vi "Puma_Ground_Control_Station_V2.0.vi"(0 "?":refnum<visa-resource-name>="COM3", 1 "?":u32=9600, 9 "XON":u8=17 format="%.0x", 14 "XOFF":u8=19 format="%.0x", 15 "?":u32=10000, 21 "?":bool=TRUE, 24 "?":u8=10 format="%.0x", 25 "bsize":u32=4096) -> ()   [LabVIEW 2015]
doc: "The Advanced Serial Read and Write example performs a Serial Port Read, a Serial Port Write, or a combination of these actions while setting some advanced serial features like buffer size, termination characters, and XON/XOFF flow control. The user selects the actions (read or write) on the front panel. If both are selected, the VI will write the data first, read the data and then close the VISA session that is opened to the port. \n\nThe parameters set for the serial port must match the parameters of the connected instrument or device. In this example, the bytes to read parameter specifies the number of bytes that the serial port reads. If there were more bytes at the port than the number specified in bytes to read, those bytes would not be read. Also, if you specify to read more bytes than the number of bytes actually read, you might receive a timeout error message.\n\nINSTRUCTIONS:\n1) Select the serial resource and configuration parameters (baud rate, data bits, parity, stop bits, flow control).\n2) Termination character can be enabled and set. Also, set the required input buffer size prior to running the example.\n3) Select the operations to be performed. \n4) Connect the serial port to your device. If no device is available, perform a loopback test by doing one of the following. Short pins 2 and 3 on a RS-232 cable or short pin 4 to pin 8 and pin 5 to pin 9 on a RS-485/422 cable. \n5) Run the VI to see the data read. (The \"read string\" will match the \"string to write\" if a loopback test was performed.)\n\nThis example exposes several advanced features that you may need for your application. Not all applications need all the features shown in this example. The input buffer size is likely an important setting that you want to control in your application. This example expands upon the flow control option for XON and XOFF, allowing the user to choose those control characters. The timeout parameter has been brought to the front panel so a user can specify the time period the VISA Read will wait for the number of bytes to read before timing out. Also, the user has several controls for the termination character, which is discussed later.\n\nNote that you can press the write and read buttons and change the bytes to read parameters on the fly, while the example is running. However, you must stop the example to change the other configuration parameters after the example has started running, and then run again.\n\nSet the I/O buffer size slightly higher the amount of data you expect to receive. This is very important for applications that don't use flow control, as you may lose characters if the receive buffer overflows.\n\nSetting the timeout period ensures that the operation returns with a timeout error if the operation cannot be performed in the specified time period. \n\nSome devices require a termination character in order to identify the end of command strings. Some devices send a termination character to signify the end of data to be read. \n\nThis example shows how you can end the Read operation once a termination character is detected in the buffer and/or append a termination character at the end of the Write data. To enable the Read to end on a termination character, use the VISA Configure Serial Port or use the VISA Properties Serial End Mode for Reads, Termination Character Enable, and Termination Character. To end the Write with a termination character, use the VISA Properties Serial End Mode for Writes, the Send End Enable, and Termination Character. In this example, the same termination character is used for both the Read and the Write. You can specify two different characters for your application, if desired.\n\nYour application may require specific characters for the XON/XOFF Flow Control. You can specify these characters with the VISA Properties Flow Control XOFF Character and Flow Control XON Character. Note that if the standard XON and XOFF characters are used, then decimal 17 and 19 are unavailable for data values. Remember that using flow control and setting an adequate buffer size allow you to prevent buffer overflows."
uses:
  <vilib>/Instr/_visa.llb/VISA Configure Serial Port (Instr).vi
panel:
  out "Numeric":i32
  out "Reset Triggered":bool
  in  "PixHawk":bool
  in  "XON 2":u8=17 format="%.0x"
  in  "XOFF 2":u8=19 format="%.0x"
  in  "?":bool=TRUE
  in  "bsize 2":u32=4096
  in  "?":u8=10 format="%.0x"
  in  "?":bool=TRUE
  in  "?":u32=10000
  in  "?":refnum<visa-resource-name>="COM3"
  in  "?":u32=9600
  out "Max Values":T1={20.764332288, 0.0, 0.0, 0.0, 0.0, 0.0, 0.0, 201.058, 25.138999999999953, 0.0, 57.16000000000008, 0.0, 8.920000000000016, 15.403999999999996}
  in  "Data Filename":string
  out "Offset 7":dbl=-251.3
  out "Multiplier 7":dbl=1.264
  out "Offset 6":dbl=-250.2
  out "Offset 5":dbl=-250.3
  out "Offset 4":dbl=-1253.0
  out "Offset 3":dbl=-250.9
  out "Offset 2":dbl=-249.8
  out "Offset 1":dbl=-251.0
  out "Multiplier 6":dbl=1.264
  out "Multiplier 5":dbl=1.277
  out "Multiplier 4":dbl=6.36
  out "Multiplier 3":dbl=1.274
  out "Multiplier 2":dbl=1.267
  out "Multiplier 1":dbl=1.277
  out "Ready to Test":bool
  out "AV5-T Open":bool
  in  "Begin Checklist":bool
  out "Manual Abort Tested":bool
  out "Flight Control On":bool
  out "Reset Triggered 2":bool
  out "Primary Safety Active":bool
  out "Craft Triggered Softkill Active":bool
  out "Hardkill Active":bool
  out "ms":dbl=163640.0
  out "vcc 6":bool
  out "gnd 6":bool=TRUE
  out "TC6":bool
  out "vcc 5":bool
  out "gnd 5":bool=TRUE
  out "TC5":bool
  out "vcc 4":bool
  out "gnd 4":bool=TRUE
  out "TC4":bool
  out "vcc 3":bool
  out "gnd 3":bool=TRUE
  out "TC3":bool
  out "vcc 2":bool
  out "gnd 2":bool=TRUE
  out "TC2":bool
  out "vcc":bool
  out "gnd":bool=TRUE
  out "TC1":bool
  out "Motor 4":dbl=1000.0
  out "Motor 3":dbl=1000.0
  out "Motor 2":dbl=1000.0
  out "Motor 1":dbl=1000.0
  out "soft kill ind":bool
  out "dump fuel ind":bool
  out "abort ind":bool
  out "run ind":bool
  out "av6-t ind":bool
  out "Control input":bool
  out "return":bool
  out "Control (on/off)":bool
  out "PT5-M":dbl=-6.084000000000003
  out "PT2-M":dbl=-10.039999999999992
  out "PT2-U":dbl=-250.3
  out "PT1-U":dbl=-38.24000000000001
  out "PT3-M":dbl=-141.336
  out "PT1-M":dbl=9.934999999999945
  out "PT4-M":dbl=181.90299999999996
  out "TC6":dbl=-2.0
  out "TC5":dbl=-2.0
  out "TC4":dbl=-2.0
  out "TC3":dbl=-2.0
  out "TC2":dbl=-2.0
  out "TC1":dbl=-2.0
  out "Output":string="h:;"
  in  "?":enum32{"Ignore", "Test"}(tab)=enum."Test"
  in  "DValve / AV6-T":bool
  in  "Flight Control Board":bool
  in  "Safety":bool
  in  "Test Run":bool
  in  "Reset Control":bool
  in  "Primary Safety":bool
  out "?":bool
  in  "Primary Safety":bool=TRUE
  in  "Soft Kill":bool
  in  "Simulate":bool
  in  "Reset FC":bool
  in  "Full Power":bool
  in  "Safety":bool=TRUE
  in  "Takeoff":bool
  in  "Calibrate":bool
  in  "abort":bool
  out "?":dbl(graph)=20.40794784
  in  "Send":bool=TRUE
  in  "Recieve":bool=TRUE
  in  "bytes to read 2":u32=1000
  out "?":u32=107
  out "?":string[](array[string])=["339", "205", "86", "191", "0", "190", "194", "-2.00", "-2.00", "-2.00", "-2.00", "-2.00", "-2.00", "555", "1000", "1000", "1000", "1000", "163640"]
  out "?":string[](array[string])=["p:339,205,86,191,0,190,194", "t:-2.00,-2.00,-2.00,-2.00,-2.00,-2.00", "v:555", "m:1000,1000,1000,1000", "h:", "s:163640", ""]
  out "?":T1(graph)={20.40794784, -2.0, -2.0, -2.0, -2.0, -2.0, -2.0, 181.90299999999996, 9.934999999999945, -141.336, -38.24000000000001, -250.3, -10.039999999999992, -6.084000000000003}
  out "Voltage Sensor":dbl=20.40794784
  in  "dump fuel":bool
  in  "?":enum32{"PT", "TC", "Motors", "Ignore"}(tab)
  in  "?":T2(tab)
  out "PT 4":dbl(graph)=-38.24000000000001
  out "PT 5":dbl(graph)=-250.3
  out "PT 2":dbl(graph)=9.934999999999945
  out "PT 6":dbl(graph)=-10.039999999999992
  out "PT 3":dbl(graph)=-141.336
  out "PT 1":dbl(graph)=181.90299999999996
  out "PT 7":dbl(graph)=-6.084000000000003
  in  "?":T3(tab)
  out "TC 1":dbl(graph)=-2.0
  out "TC 2":dbl(graph)=-2.0
  out "TC 3":dbl(graph)=-2.0
  out "TC 4":dbl(graph)=-2.0
  out "TC 5":dbl(graph)=-2.0
  out "TC 6":dbl(graph)=-2.0
  out "Motors":cluster{dbl, dbl, dbl, dbl}(graph)={1000.0, 1000.0, 1000.0, 1000.0}
  out "?":bool=TRUE
  out "String":string
  in  "String 3":string
  in  "?":bool=TRUE
  in  "tank iso":bool
  in  "Av-6Tt":bool
  in  "FC-U Toggle":bool
  in  "FOU":bool
  out "AV4-T":bool
  out "AV3-T":bool
  out "AV2-T":bool
  out "AV1-T":bool
  out "AV6-T":bool
  out "AV5-T":bool
  out "FO-U":bool
  out "FC-U":bool
  out "?":dbl(slide) scale=0.2..200.0
  # "green=open - check thermocouple attachments\nred=short gnd - contact Power or GNC\nblue=short vcc - contact Power or GNC"
  # "String Parsing Indicator"
  # "Data From Craft:"
  # "FC-U"
  # "FO-U"
  # "receive"
  # "AV1-M"
  # "AV2-M"
  # "AV3-M"
  # "AV4-M"
  # "AV5-T"
  # "send"
  # "AV6-T"
  # "Voltage"
  # "TCp2-M"
  # "Tcw1-E"
  # "TCp1-M"
  # "TCw4-E"
  # "TCw3-E"
  # "TCw2-E"
  # "PT4-M"
  # "PT1-M"
  # "PT3-M"
  # "PT1-U"
  # "PT2-U"
  # "PT2-M"
  # "PT5-M"
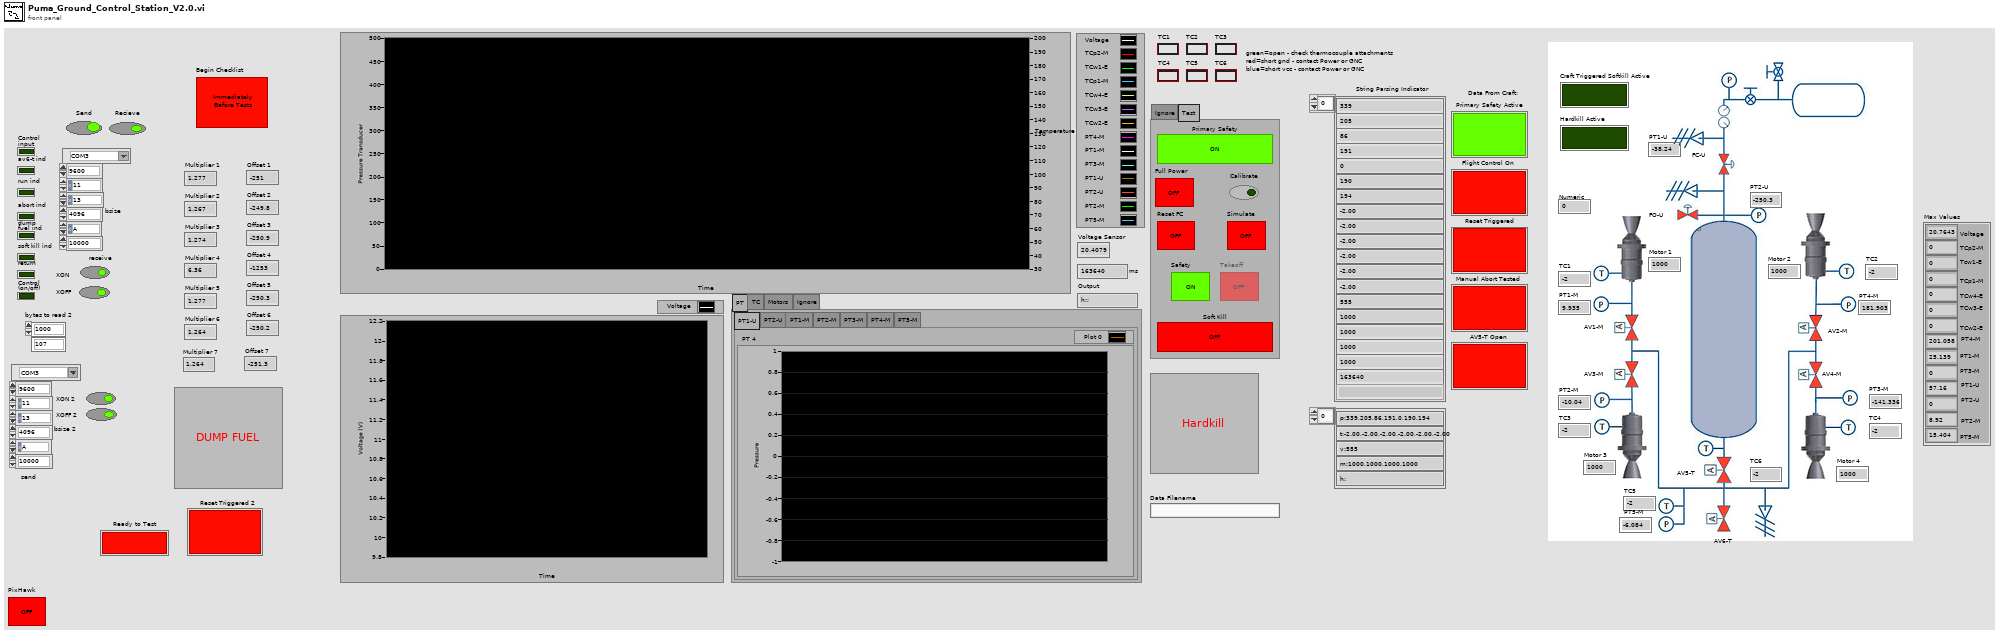
[diagram p1: front panel]
types:
  T1 = cluster{dbl, dbl, dbl, dbl, dbl, dbl, dbl, dbl, dbl, dbl, dbl, dbl, dbl, dbl}
  T2 = enum32{"PT1-U", "PT2-U", "PT1-M", "PT2-M", "PT3-M", "PT4-M", "PT5-M"}
  T3 = enum32{"TCp2-M", "TCw1-E", "TCp1-M", "TCw4-E", "TCw3-E", "TCw2-E"}
  T4 = enum16{"open", "replace", "create", "open or create", "replace or create", "replace or create with confirmation"}
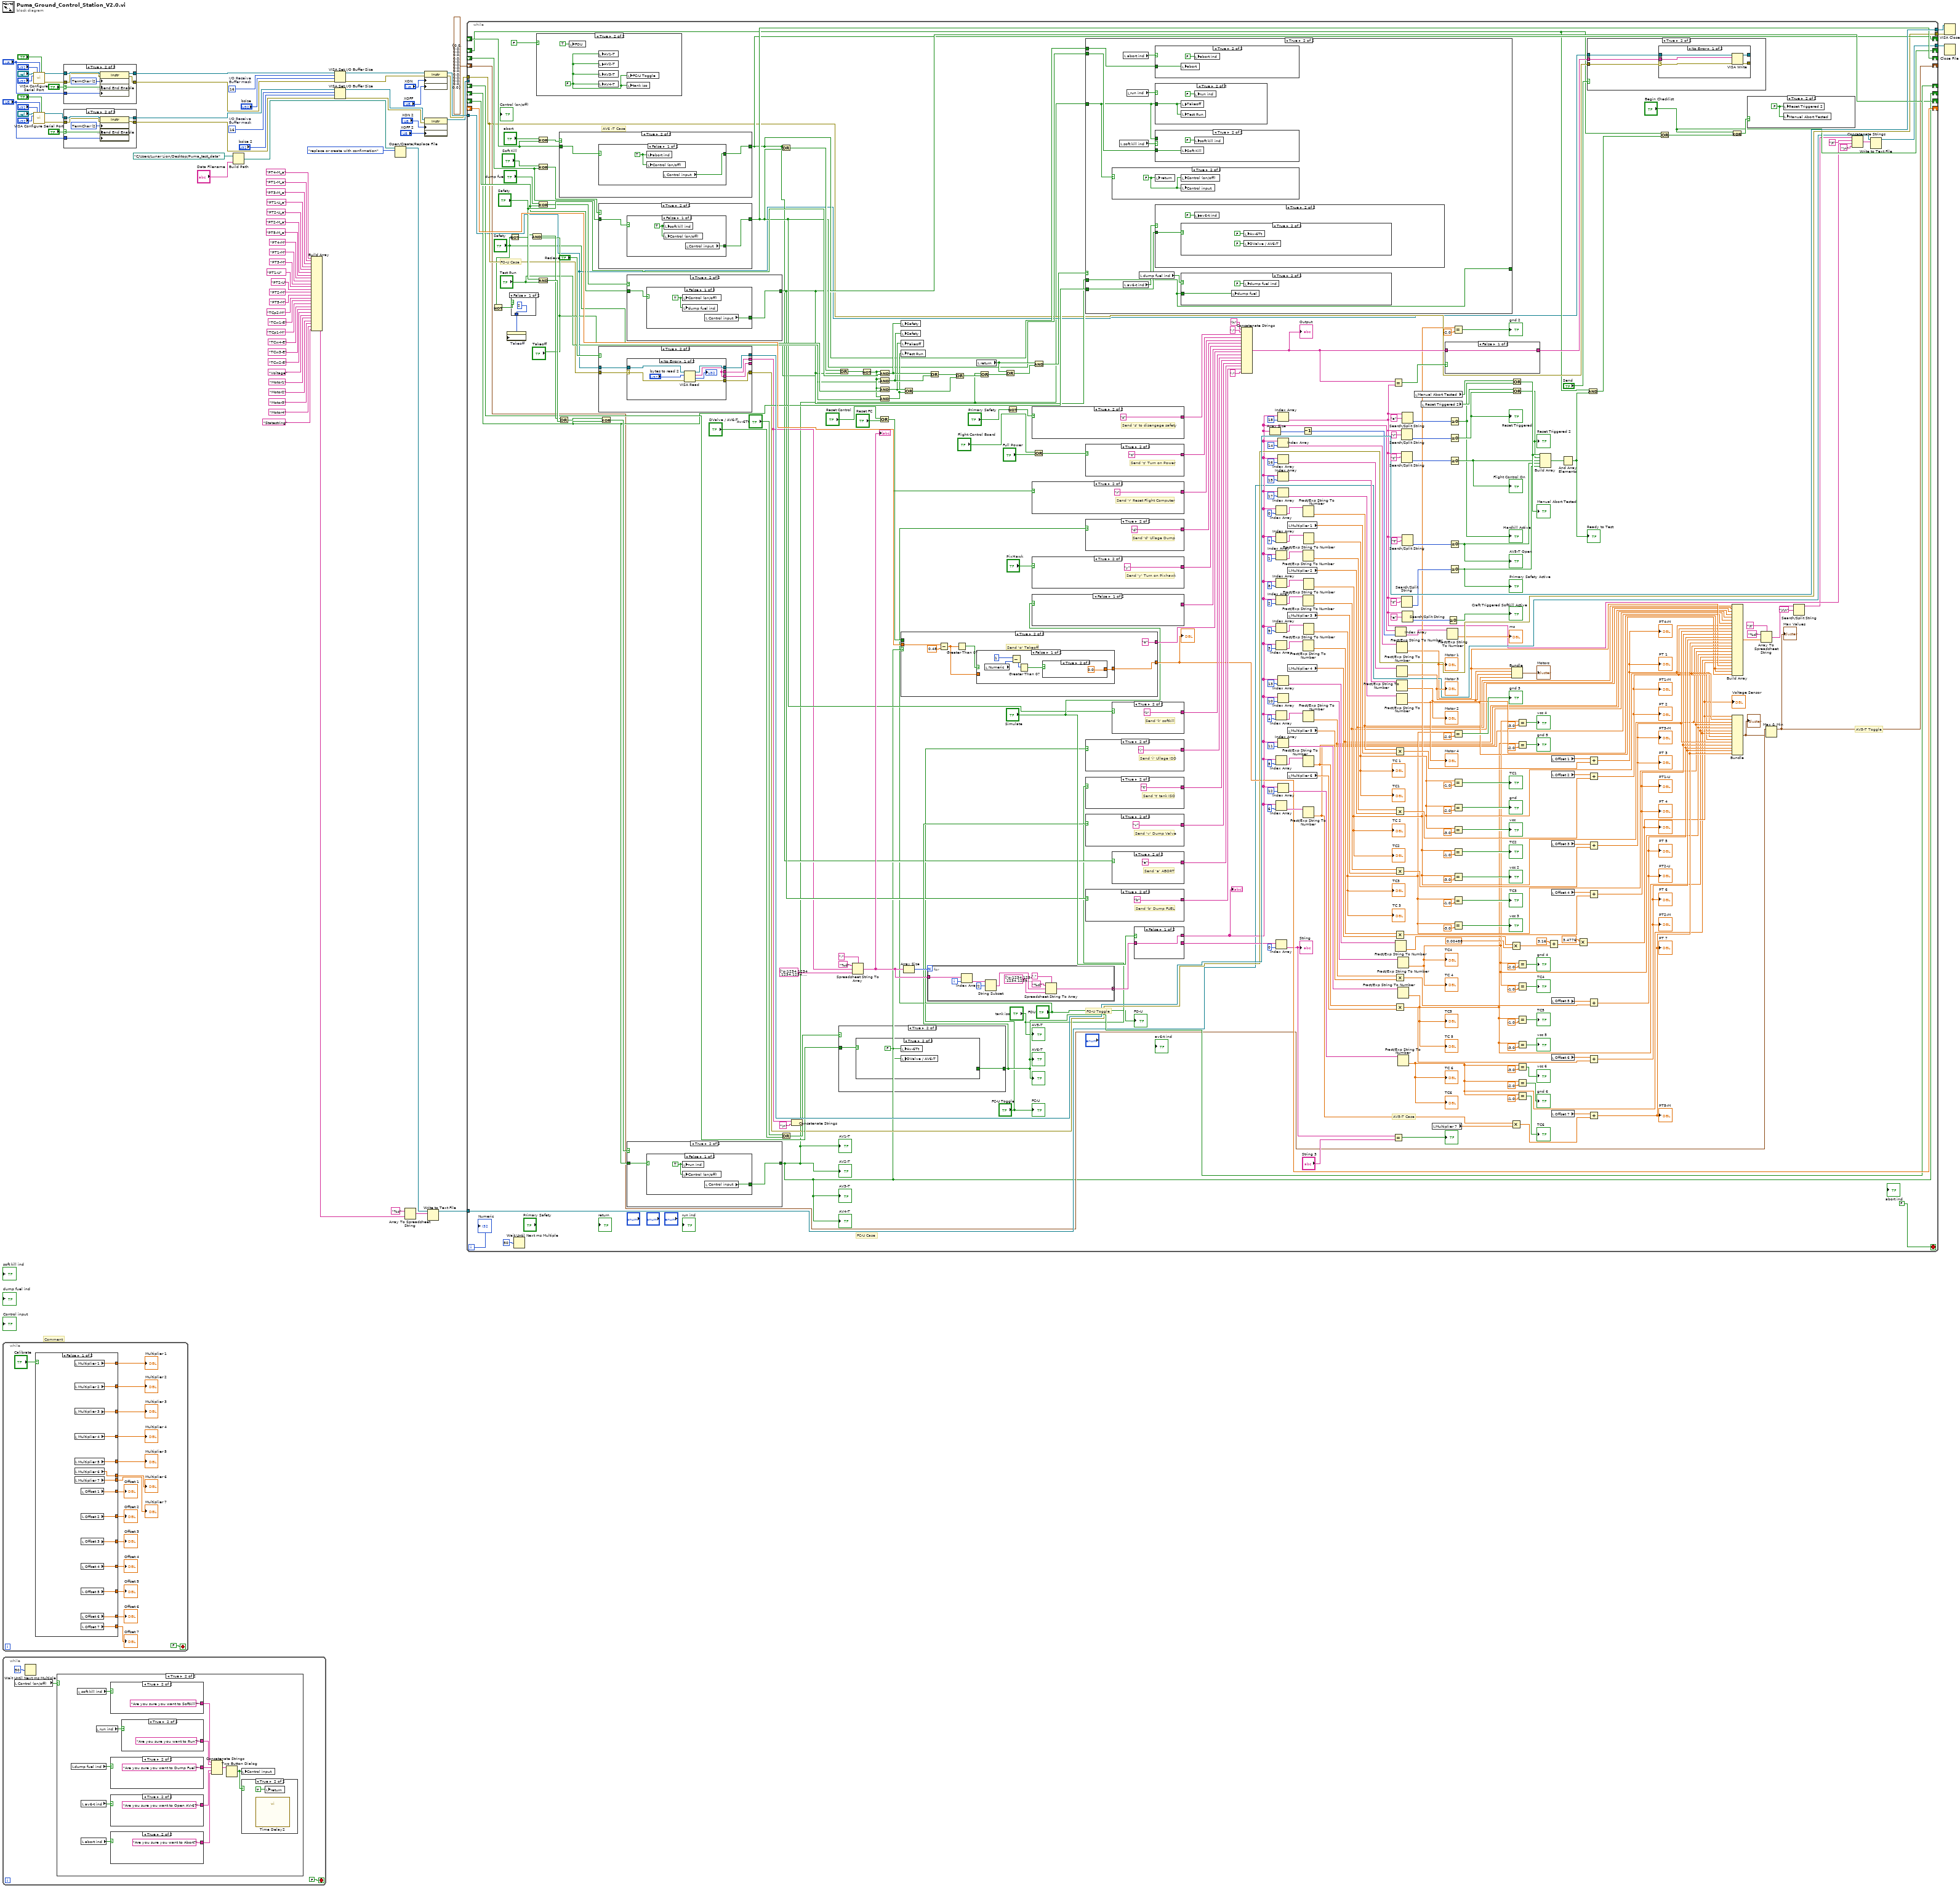
[diagram p0: block diagram]
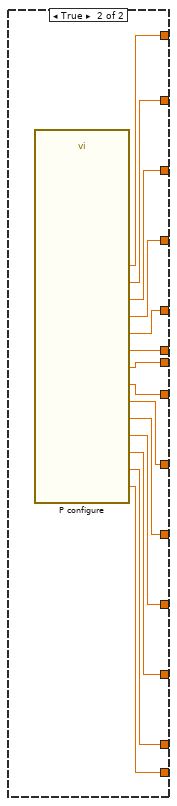
[diagram p3: hidden frame]
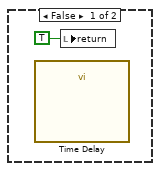
[diagram p10: hidden frame]
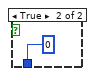
[diagram p11: hidden frame]
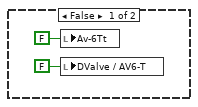
[diagram p17: hidden frame]
diagram:
  w45 = u16 16  # I/O Receive Buffer mask
  w70 = u16 16  # I/O Receive Buffer mask
  # "Comment"
  n1 = while {
    stop <- FALSE stop-if-true
    n2 = case shown="False" "Calibrate" {
      tunnel: [w104 w118] -> w88
      tunnel: [w103 w117] -> w87
      tunnel: [w102 w116] -> w86
      tunnel: [w101 w115] -> w85
      tunnel: [w100 w114] -> w84
      tunnel: [w99 w113] -> w83
      tunnel: [w98 w112] -> w82
      tunnel: [w96 w111] -> w81
      tunnel: [w97 w110] -> w80
      tunnel: [w95 w109] -> w79
      tunnel: [w94 w108] -> w78
      tunnel: [w93 w107] -> w77
      tunnel: [w92 w106] -> w76
      tunnel: [w91 w105] -> w75
      frame False {
        n3 = local read "Multiplier 1"() -> (w104:dbl)
        n4 = local read "Multiplier 2"() -> (w103:dbl)
        n5 = local read "Multiplier 3"() -> (w102:dbl)
        n6 = local read "Multiplier 4"() -> (w101:dbl)
        n7 = local read "Multiplier 5"() -> (w100:dbl)
        n8 = local read "Multiplier 6"() -> (w99:dbl)
        n9 = local read "Multiplier 7"() -> (w98:dbl)
        n10 = local read "Offset 1"() -> (w96:dbl)
        n11 = local read "Offset 2"() -> (w97:dbl)
        n12 = local read "Offset 3"() -> (w95:dbl)
        n13 = local read "Offset 4"() -> (w94:dbl)
        n14 = local read "Offset 5"() -> (w93:dbl)
        n15 = local read "Offset 6"() -> (w92:dbl)
        n16 = local read "Offset 7"() -> (w91:dbl)
      }
      frame True {
        n17 = call "P configure.vi"() -> ("Multiplier 1"=w118:dbl, "Offset 1"=w111:dbl, "Multiplier 2"=w117:dbl, "Offset 2"=w110:dbl, "Multiplier 3"=w116:dbl, "Offset 6"=w106:dbl, "Offset 3"=w109:dbl, "Offset 7"=w105:dbl, "Multiplier 4"=w115:dbl, "Multiplier 7"=w112:dbl, "Multiplier 6"=w113:dbl, "Offset 5"=w107:dbl, "Multiplier 5"=w114:dbl, "Offset 4"=w108:dbl)  [unwired: 2 in]
      }
    }
    "Multiplier 1" <- w88
    "Multiplier 2" <- w87
    "Multiplier 3" <- w86
    "Multiplier 4" <- w85
    "Multiplier 5" <- w84
    "Offset 1" <- w81
    "Offset 2" <- w80
    "Offset 3" <- w79
    "Offset 4" <- w78
    "Offset 5" <- w77
    "Offset 6" <- w76
    "Multiplier 7" <- w82
    "Offset 7" <- w75
    "Multiplier 6" <- w83
  }
  n18 = while {
    stop <- FALSE stop-if-true
    n19 = local read "Control (on/off)"() -> (w121:bool)
    n20 = Wait Until Next ms Multiple(millisecond multiple=u32 50 ("milliseconds to wait")) -> ()  [unwired: 1 out]
    n21 = case shown="True" w121 {
      frame False {
      }
      frame True {
        n22 = local read "dump fuel ind"() -> (w130:bool)
        n23 = local read "soft kill ind"() -> (w128:bool)
        n24 = local read "av6-t ind"() -> (w131:bool)
        n25 = local read "abort ind"() -> (w132:bool)
        n26 = local read "run ind"() -> (w129:bool)
        n27 = case shown="True" w128 {
          tunnel: [_ "Are you sure you want to Softkill?"] -> w123
          frame False {
          }
          frame True {
          }
        }
        n28 = case shown="True" w130 {
          tunnel: [_ "Are you sure you want to Dump Fuel?"] -> w125
          frame False {
          }
          frame True {
          }
        }
        n29 = case shown="True" w131 {
          tunnel: [_ "Are you sure you want to Open AV-6?"] -> w126
          frame False {
          }
          frame True {
          }
        }
        n30 = case shown="True" w132 {
          tunnel: [_ "Are you sure you want to Abort?"] -> w127
          frame False {
          }
          frame True {
          }
        }
        n31 = case shown="True" w129 {
          tunnel: [_ "Are you sure you want to Run?"] -> w124
          frame False {
          }
          frame True {
          }
        }
        n32 = Concatenate Strings(w123, w124, w125, w126, w127) -> (w122:string)
        n33 = Two Button Dialog(message=w122) -> (T button?=w133:bool)  [unwired: 2 in]
        n34 = local write "Control input"(w133) -> ()
        n35 = case shown="True" w133 {
          frame False {
            n36 = call "Time Delay"() -> ()  [unwired: 11 in, 1 out]
            n37 = local write "return"(TRUE) -> ()
          }
          frame True {
            n38 = call "Time Delay2"() -> ()  [unwired: 11 in, 1 out]
            n39 = local write "return"(TRUE) -> ()
          }
        }
      }
    }
  }
  n40 = call-poly "VISA Configure Serial Port"("VISA resource name"="?", "timeout (10sec)"="?", "termination char\n(0xA = '\\n' = LF)"="?", "Enable Termination\nChar (T)"="?", "baud rate (9600)"="?") -> ("VISA resource name out"=w59:refnum<visa-resource-name>, "error out"=w62:errorcluster)  [unwired: 5 in, 4 out]
  n41 = call-poly "VISA Configure Serial Port"("VISA resource name"="?", "timeout (10sec)"="?", "termination char\n(0xA = '\\n' = LF)"="?", "Enable Termination\nChar (T)"="?", "baud rate (9600)"="?") -> ("VISA resource name out"=w34:refnum<visa-resource-name>, "error out"=w37:errorcluster)  [unwired: 5 in, 4 out]
  n42 = case shown="True" "?" {
    selector: "?" -> [_ w143]
    tunnel: w59 -> [w141 w149]
    tunnel: w62 -> [w142 w148]
    tunnel: [w141 w147] -> w60
    tunnel: [w142 w146] -> w61
    tunnel: "?" -> [_ w144]
    frame False {
    }
    frame True {
      w145 = u16 2 items=["None", "LastBit", "TermChar", "Break"] ("Serial Settings:Serial End Mode for Writes")
      n43 = property class="Instr"(reference=w149, error in=w148, "Serial Settings:End Mode for Writes"=w145, "Message Based Settings:Send End Enable"=w143, "Message Based Settings:Termination Character"=w144) -> (reference out=w147:refnum<visa-resource-name>, error out=w146:errorcluster)
    }
  }
  n44 = case shown="True" "?" {
    selector: "?" -> [_ w152]
    tunnel: w34 -> [w150 w158]
    tunnel: w37 -> [w151 w157]
    tunnel: [w150 w156] -> w35
    tunnel: [w151 w155] -> w36
    tunnel: "?" -> [_ w153]
    frame False {
    }
    frame True {
      w154 = u16 2 items=["None", "LastBit", "TermChar", "Break"] ("Serial Settings:Serial End Mode for Writes")
      n45 = property class="Instr"(reference=w158, error in=w157, "Serial Settings:End Mode for Writes"=w154, "Message Based Settings:Send End Enable"=w152, "Message Based Settings:Termination Character"=w153) -> (reference out=w156:refnum<visa-resource-name>, error out=w155:errorcluster)
    }
  }
  n46 = Build Path(base path=path "C:/Users/Lunar Lion/Desktop/Puma_test_data" ("file path (use dialog)"), name or relative path="Data Filename") -> (appended path=w53:path)
  n47 = Build Array("PT4-M_a", "PT1-M_a", "PT3-M_a", "PT1-U_a", "PT2-U_a", "PT2-M_a", "PT5-M_a", "PT4-M", "PT1-M", "PT3-M", "PT1-U", "PT2-U", "PT2-M", "PT5-M", "TCp2-M", "TCw1-E", "TCp1-M", "TCw4-E", "TCw3-E", "TCw2-E", "Voltage", "Motor1", "Motor2", "Motor3", "Motor4", "Statestring") -> (w6:string[])
  n48 = VISA Set I/O Buffer Size(VISA resource name=w60, mask (16)=w70, size (4096)="bsize", error in (no error)=w61) -> (VISA resource name out=w66:refnum<visa-resource-name>, error out=w65:errorcluster)
  n49 = VISA Set I/O Buffer Size(VISA resource name=w35, mask (16)=w45, size (4096)="bsize 2", error in (no error)=w36) -> (VISA resource name out=w41:refnum<visa-resource-name>, error out=w40:errorcluster)
  n50 = Open/Create/Replace File(file path (use dialog)=w53, operation (0:open)=T4."replace or create with confirmation") -> (refnum out=w3:refnum<file>)  [unwired: 4 in, 2 out]
  n51 = Array To Spreadsheet String(array=w6, 3:"%s" ("format string")) -> (spreadsheet string=w4:string)  [unwired: 1 in]
  n52 = property class="Instr"(reference=w66, error in=w65, "Serial Settings:Flow Control XON Character"="XON", "Serial Settings:Flow Control XOFF Character"="XOFF") -> (reference out=w58:refnum<visa-resource-name>, error out=w57:errorcluster)
  n53 = property class="Instr"(reference=w41, error in=w40, "Serial Settings:Flow Control XON Character"="XON 2", "Serial Settings:Flow Control XOFF Character"="XOFF 2") -> (reference out=w33:refnum<visa-resource-name>)  [unwired: 1 out]
  n54 = Write to Text File(file (use dialog)=w3, text=w4) -> (refnum out=w2:refnum<file>)  [unwired: 2 in, 2 out]
  n55 = while {
    tunnel: w58 -> [w187]
    tunnel: w57 -> [w267]
    tunnel: [w403] -> w1
    tunnel: [w329] -> w56
    shift-right: [w375] -> _
    shift-left: _ -> [w374]
    shift-right: [w186] -> _
    shift-left: _ -> [w333]
    shift-right: [w341] -> _
    shift-left: _ -> [w342]
    shift-right: [w331] -> _
    shift-left: _ -> [w357]
    shift-right: [w332] -> _
    shift-left: _ -> [w354]
    shift-right: [w334] -> _
    shift-left: _ -> [w337]
    shift-right: ["Begin Checklist"] -> _
    shift-left: _ -> [w248]
    tunnel: w2 -> [w220]
    tunnel: [w217] -> w52
    shift-right: [w190] -> _
    shift-left: T1 {0.0, 0.0, 0.0, 0.0, 0.0, 0.0, 0.0, 0.0, 0.0, 0.0, 0.0, 0.0, 0.0, 0.0} -> [w189]
    tunnel: w33 -> [_]
    i -> [w159]
    stop <- FALSE stop-if-true
    # "FO-U Case"
    # "AV6 -T Case"
    # "AV5-T Case"
    # "FC-U Case"
    # "FO-U Toggle"
    # "AV5-T Toggle"
    n56 = Not(x="Safety") -> (.not. x?=w162:bool)
    n57 = Not(x="Safety") -> (.not. x?=w160:bool)
    n58 = case shown="False" w162 {
      tunnel: [2 0] -> w161
      frame False {
      }
      frame True {
      }
    }
    n59 = property on="Takeoff" class="Bool (strict)"("DisabledEnum"=w161) -> ()  [unwired: 2 in, 2 out]
    n60 = Wait Until Next ms Multiple(millisecond multiple=u32 50 ("milliseconds to wait")) -> ()  [unwired: 1 out]
    n61 = And(x=w160, y="Takeoff") -> (x .and. y?=w389:bool)
    n62 = case shown="True" FALSE {
      frame False {
      }
      frame True {
        w437 = FALSE
        n63 = local write "FOU"(TRUE) -> ()
        n64 = local write "AV1-T"(w437) -> ()
        n65 = local write "AV2-T"(w437) -> ()
        n66 = local write "AV3-T"(w437) -> ()
        n67 = local write "AV4-T"(w437) -> ()
        n68 = local write "FC-U Toggle"(w437) -> ()
        n69 = local write "tank iso"(w437) -> ()
      }
    }
    n70 = Exclusive Or(1:w357, 2:"abort") -> (0:w359:bool)
    n71 = Exclusive Or(1:w337, 2:"Soft Kill") -> (0:w335:bool)
    n72 = Exclusive Or(1:w354, 2:"dump fuel") -> (0:w356:bool)
    n73 = And(x="Safety", y="Test Run") -> (x .and. y?=w390:bool)
    n74 = Or(x=w389, y=w390) -> (x .or. y?=w362:bool)
    n75 = case shown="True" w359 {
      tunnel: [w483 w485] -> w331
      tunnel: w357 -> [w483 w484]
      frame False {
      }
      frame True {
        n76 = case shown="False" w484 {
          tunnel: [w486 FALSE ("T button?")] -> w485
          frame False {
            w487 = TRUE
            n77 = local write "abort ind"(w487) -> ()
            n78 = local write "Control (on/off)"(w487) -> ()
            n79 = local read "Control input"() -> (w486:bool)
          }
          frame True {
          }
        }
      }
    }
    n80 = case shown="True" w335 {
      tunnel: [w473 w475] -> w334
      tunnel: w337 -> [w473 w474]
      frame False {
      }
      frame True {
        n81 = case shown="False" w474 {
          tunnel: [w476 _] -> w475
          frame False {
            w477 = TRUE
            n82 = local write "soft kill ind"(w477) -> ()
            n83 = local write "Control (on/off)"(w477) -> ()
            n84 = local read "Control input"() -> (w476:bool)
          }
          frame True {
          }
        }
      }
    }
    n85 = case shown="True" "Recieve" {
      tunnel: w267 -> [w537 w542]
      tunnel: w187 -> [w538 w541]
      tunnel: [w537 w544] -> w329
      tunnel: [w538 w543] -> w403
      tunnel: [_ w540] -> _
      tunnel: [_ w539] -> w219
      frame False {
      }
      frame True {
        n86 = case "Read bytes from port." shown="No Error" w542 {
          selector: w542 -> [w547 w552]
          tunnel: [w550 w552] -> w544
          tunnel: [w551 w553] -> w543
          tunnel: w541 -> [w548 w553]
          tunnel: [w545 _] -> w540
          tunnel: [w545 _] -> w539
          frame No Error {
            n87 = VISA Read(VISA resource name=w548, byte count="bytes to read 2", error in (no error)=w547) -> (VISA resource name out=w551:refnum<visa-resource-name>, read buffer=w545:string, return count=→"?":u32, error out=w550:errorcluster)
          }
          frame Error {
            # "Error occurred \nreading Bytes at \nSerial Port"
          }
        }
      }
    }
    n88 = Exclusive Or(1:w333, 2:w362) -> (0:w361:bool)
    n89 = case shown="True" w356 {
      tunnel: [w478 w480] -> w332
      tunnel: w354 -> [w478 w479]
      frame False {
      }
      frame True {
        n90 = case shown="False" w479 {
          tunnel: [w482 _] -> w480
          frame False {
            w481 = TRUE
            n91 = local write "Control (on/off)"(w481) -> ()
            n92 = local write "dump fuel ind"(w481) -> ()
            n93 = local read "Control input"() -> (w482:bool)
          }
          frame True {
          }
        }
      }
    }
    n94 = case shown="True" w361 {
      tunnel: [w489 w491] -> w186
      tunnel: w333 -> [w489 w490]
      frame False {
      }
      frame True {
        n95 = case shown="False" w490 {
          tunnel: [w493 _] -> w491
          frame False {
            w492 = TRUE
            n96 = local write "run ind"(w492) -> ()
            n97 = local write "Control (on/off)"(w492) -> ()
            n98 = local read "Control input"() -> (w493:bool)
          }
          frame True {
            w494 = FALSE
            n99 = local write "Test Run"(w494) -> ()
            n100 = local write "Control (on/off)"(w494) -> ()
            n101 = local write "Takeoff"(w494) -> ()
          }
        }
      }
    }
    "AV1-T" <- w186
    "AV4-T" <- w186
    "AV2-T" <- w186
    "AV3-T" <- w186
    n102 = Or(x=w331, y=w334) -> (x .or. y?=w360:bool)
    n103 = Or(x="Av-6Tt", y="DValve / AV6-T") -> (x .or. y?=w338:bool)
    n104 = Concatenate Strings(w219, "\n" ("string")) -> ()  [unwired: 1 out]
    n105 = Or(x=w360, y=w332) -> (x .or. y?=w326:bool)
    n106 = case shown="True" w338 {
      tunnel: [w467 w468] -> w341
      tunnel: w342 -> [w467 w469]
      frame False {
      }
      frame True {
        n107 = case shown="True" w469 {
          tunnel: [w471 _] -> w468
          frame False {
            w470 = TRUE
            n108 = local write "Control (on/off)"(w470) -> ()
            n109 = local write "av6-t ind"(w470) -> ()
            n110 = local read "Control input"() -> (w471:bool)
          }
          frame True {
            w472 = FALSE
            n111 = local write "Av-6Tt"(w472) -> ()
            n112 = local write "DValve / AV6-T"(w472) -> ()
          }
        }
      }
    }
    "AV6-T" <- w341
    "?" <- w341
    n113 = Spreadsheet String To Array(delimiter (Tab)=";", format string="%d", spreadsheet string=w219, array type (2D Dbl)=string[] ["p:1234.1234.1234.1234,1234,1234", "t:1234,1234,1234"] ("Array of Strings 3")) -> (array=w429:string[])
    "?" <- w429
    n114 = Not(x=w326) -> (.not. x?=w364:bool)
    n115 = Or(x="Reset Control", y="Reset FC") -> (x .or. y?=w376:bool)
    n116 = And(x=w364, y="Safety") -> (x .and. y?=w346:bool)
    n117 = And(x=w364, y="Safety") -> (x .and. y?=w345:bool)
    n118 = And(x=w364, y="Takeoff") -> (x .and. y?=w344:bool)
    n119 = And(x=w364, y="Test Run") -> (x .and. y?=w343:bool)
    n120 = local write "Safety"(w346) -> ()
    n121 = local write "Safety"(w345) -> ()
    n122 = local write "Takeoff"(w344) -> ()
    n123 = local write "Test Run"(w343) -> ()
    n124 = case shown="True" w186 {
      tunnel: [_ "o" ("write buffer")] -> w394
      tunnel: w374 -> [w506 w514]
      tunnel: [w507 w510] -> w375
      tunnel: w376 -> [w505 _]
      frame False {
        n125 = case shown="False" w505 {
          tunnel: [w508 200.0] -> w507
          tunnel: w506 -> [w508 _]
          frame False {
          }
          frame True {
          }
        }
      }
      frame True {
        # "Send 'o' Takeoff"
        n126 = Subtract(x=w514, y=0.48) -> (x-y=w511:dbl)
        n127 = Greater Than 0?(x=w511) -> (x > 0?=w512:bool)
        n128 = case shown="False" w512 {
          tunnel: w511 -> [_ w523]
          tunnel: [w518 w523] -> w510
          frame False {
            n129 = local read "Numeric"() -> (w520:i32)
            n130 = Subtract(x=1, y=w520) -> (x-y=w517:i32)
            n131 = Greater Than 0?(x=w517) -> (x > 0?=w519:bool)
            n132 = case shown="True" w519 {
              tunnel: [200.0 0.0] -> w518
              frame False {
              }
              frame True {
              }
            }
          }
          frame True {
          }
        }
      }
    }
    "?" <- w375
    n133 = Or(x=w344, y=w343) -> (x .or. y?=w348:bool)
    n134 = Array Size(array=w429) -> (size(s)=w430:i32)
    n135 = for {
      N: w430 -> [_]
      tunnel: w429 -> [w562]
      tunnel: [w554] -> w372 mode=concatenating
      i -> [w561]
      n136 = Index Array(array=w562, index=w561) -> (element=w557:string)
      n137 = String Subset(string=w557, offset (0)=2) -> (substring=w555:string)  [unwired: 1 in]
      n138 = Spreadsheet String To Array(delimiter (Tab)=",", format string="%d", spreadsheet string=w555, array type (2D Dbl)=string[] ["p:1234.1234.1234.1234,1234,1234", "t:1234,1234,1234"] ("Array of Strings 3")) -> (array=w554:string[])
    }
    n139 = Or(x=w346, y=w345) -> (x .or. y?=w349:bool)
    n140 = Or(x=w349, y=w348) -> (x .or. y?=w347:bool)
    n141 = local read "return"() -> (w352:bool)
    n142 = Or(x=w186, y=w347) -> (x .or. y?=w350:bool)
    n143 = Or(x=w352, y=w350) -> (x .or. y?=w353:bool)
    n144 = Not(x="Primary Safety") -> (.not. x?=w164:bool)
    n145 = case shown="True" w164 {
      tunnel: [_ "s" ("write buffer")] -> w400
      frame False {
      }
      frame True {
        # "Send 's' to disengage safety"
      }
    }
    n146 = case shown="True" w376 {
      tunnel: [_ "r" ("write buffer")] -> w398
      frame False {
      }
      frame True {
        # "Send 'r' Reset Flight Computer"
      }
    }
    n147 = case shown="True" "PixHawk" {
      tunnel: [_ "y" ("write buffer")] -> w396
      frame False {
      }
      frame True {
        # "Send 'y' Turn on Pixhawk"
      }
    }
    n148 = case shown="False" "Simulate" {
      tunnel: [_ "p" ("write buffer")] -> w395
      frame False {
      }
      frame True {
        # "Send 'p' begin flight profile sim"
      }
    }
    n149 = Or(x="Flight Control Board", y="Full Power") -> (x .or. y?=w386:bool)
    n150 = And(x=w352, y=w353) -> (x .and. y?=w351:bool)
    n151 = case shown="True" w351 {
      tunnel: w186 -> [_ w442]
      tunnel: w334 -> [_ w445]
      tunnel: w333 -> [_ w444]
      tunnel: [_ w443] -> _
      tunnel: w332 -> [_ w443]
      tunnel: w331 -> [_ w441]
      frame False {
      }
      frame True {
        n152 = case shown="True" w442 {
          frame False {
            w465 = FALSE
            n153 = local write "return"(w465) -> ()
            n154 = local write "Control (on/off)"(w465) -> ()
            n155 = local write "Control input"(w465) -> ()
          }
          frame True {
            w466 = FALSE
            n156 = local write "return"(w466) -> ()
            n157 = local write "Control (on/off)"(w466) -> ()
            n158 = local write "Control input"(w466) -> ()
          }
        }
        n159 = local read "soft kill ind"() -> (w450:bool)
        n160 = local read "abort ind"() -> (w447:bool)
        n161 = local read "av6-t ind"() -> (w446:bool)
        n162 = local read "run ind"() -> (w448:bool)
        n163 = local read "dump fuel ind"() -> (w449:bool)
        n164 = case shown="True" w447 {
          tunnel: w441 -> [_ w457]
          frame False {
          }
          frame True {
            n165 = local write "abort"(w457) -> ()
            n166 = local write "abort ind"(FALSE) -> ()
          }
        }
        n167 = case shown="True" w448 {
          tunnel: w442 -> [_ w464]
          frame False {
          }
          frame True {
            n168 = local write "Takeoff"(w464) -> ()
            n169 = local write "Test Run"(w464) -> ()
            n170 = local write "run ind"(FALSE) -> ()
          }
        }
        n171 = case shown="True" w450 {
          tunnel: w442 -> [_ _]
          tunnel: w445 -> [_ w459]
          frame False {
          }
          frame True {
            n172 = local write "Soft Kill"(w459) -> ()
            n173 = local write "soft kill ind"(FALSE) -> ()
          }
        }
        n174 = case shown="True" w446 {
          tunnel: w444 -> [_ w452]
          frame False {
          }
          frame True {
            n175 = case shown="True" w452 {
              frame False {
                n176 = local write "Av-6Tt"(FALSE) -> ()
                n177 = local write "DValve / AV6-T"(FALSE) -> ()
              }
              frame True {
                n178 = local write "Av-6Tt"(FALSE) -> ()
                n179 = local write "DValve / AV6-T"(FALSE) -> ()
              }
            }
            n180 = local write "av6-t ind"(FALSE) -> ()
          }
        }
        n181 = case shown="True" w449 {
          tunnel: w443 -> [_ w461]
          frame False {
          }
          frame True {
            n182 = local write "dump fuel"(w461) -> ()
            n183 = local write "dump fuel ind"(FALSE) -> ()
          }
        }
      }
    }
    n184 = case shown="True" w386 {
      tunnel: [_ "z" ("write buffer")] -> w399
      frame False {
      }
      frame True {
        # "Send 'z' Turn on Power"
      }
    }
    n185 = case shown="True" "FOU" {
      tunnel: [_ "d" ("write buffer")] -> w385
      frame False {
      }
      frame True {
        # "Send 'd' Ullage Dump"
      }
    }
    n186 = case shown="True" "FC-U Toggle" {
      tunnel: [_ "i" ("write buffer")] -> w384
      frame False {
      }
      frame True {
        # "Send 'i' Ullage ISO"
      }
    }
    n187 = case shown="True" "tank iso" {
      tunnel: [_ "t" ("write buffer")] -> w383
      frame False {
      }
      frame True {
        # "Send 't' tank ISO"
      }
    }
    n188 = case shown="True" w341 {
      tunnel: [_ "v" ("write buffer")] -> w382
      frame False {
      }
      frame True {
        # "Send 'v' Dump Valve"
      }
    }
    n189 = case shown="True" w332 {
      tunnel: [_ "b" ("write buffer")] -> w381
      frame False {
      }
      frame True {
        # "Send 'b' Dump FUEL"
      }
    }
    n190 = case shown="True" w334 {
      tunnel: [_ "k" ("write buffer")] -> w397
      frame False {
      }
      frame True {
        # "Send 'k' softkill"
      }
    }
    n191 = case shown="True" w331 {
      tunnel: [_ "a" ("write buffer")] -> w380
      frame False {
      }
      frame True {
        # "Send 'a' ABORT"
      }
    }
    n192 = case shown="False" "Simulate" {
      tunnel: w372 -> [w495 w496]
      tunnel: [w495 w496] -> w271
      tunnel: [_ w496] -> w371
      frame False {
      }
      frame True {
      }
    }
    "?" <- w271
    n193 = Concatenate Strings("h" ("string"), ":" ("string"), w400, w399, w398, w385, w396, w395, w394, w397, w384, w383, w382, w380, w381, ";" ("string")) -> (w321:string)
    "Output" <- w321
    n194 = Array Size(array=w271) -> (size(s)=w270:i32)
    n195 = Index Array(array=w271, index=0) -> (element=w422:string)
    n196 = Index Array(array=w271, index=7) -> (element=w411:string)
    n197 = Index Array(array=w271, index=1) -> (element=w421:string)
    n198 = Index Array(array=w271, index=8) -> (element=w410:string)
    n199 = Index Array(array=w271, index=2) -> (element=w420:string)
    n200 = Index Array(array=w271, index=9) -> (element=w409:string)
    n201 = Index Array(array=w271, index=3) -> (element=w419:string)
    n202 = Index Array(array=w271, index=4) -> (element=w418:string)
    n203 = Index Array(array=w271, index=5) -> (element=w417:string)
    n204 = Index Array(array=w271, index=6) -> (element=w378:string)
    n205 = Index Array(array=w371, index=0) -> (element=w370:string)
    "String" <- w370
    n206 = Index Array(array=w271, index=18) -> (element=w201:string)
    n207 = Index Array(array=w271, index=14) -> (element=w316:string)
    n208 = Index Array(array=w271, index=16) -> (element=w314:string)
    n209 = Index Array(array=w271, index=15) -> (element=w315:string)
    n210 = Index Array(array=w271, index=17) -> (element=w313:string)
    n211 = Index Array(array=w271, index=13) -> (element=w401:string)
    n212 = Index Array(array=w271, index=10) -> (element=w407:string)
    n213 = Index Array(array=w271, index=11) -> (element=w406:string)
    n214 = Index Array(array=w271, index=12) -> (element=w405:string)
    n215 = local read "Multiplier 1"() -> (w235:dbl)
    n216 = local read "Multiplier 2"() -> (w233:dbl)
    n217 = local read "Multiplier 3"() -> (w231:dbl)
    n218 = local read "Multiplier 4"() -> (w229:dbl)
    n219 = local read "Multiplier 5"() -> (w227:dbl)
    n220 = local read "Multiplier 6"() -> (w224:dbl)
    n221 = Decrement(x=w270) -> (x-1=w269:i32)
    n222 = Fract/Exp String To Number(string=w422) -> (number=w197:dbl)  [unwired: 3 in, 1 out]
    n223 = Fract/Exp String To Number(string=w421) -> (number=w196:dbl)  [unwired: 3 in, 1 out]
    n224 = Fract/Exp String To Number(string=w420) -> (number=w195:dbl)  [unwired: 3 in, 1 out]
    n225 = Fract/Exp String To Number(string=w419) -> (number=w194:dbl)  [unwired: 3 in, 1 out]
    n226 = Fract/Exp String To Number(string=w418) -> (number=w193:dbl)  [unwired: 3 in, 1 out]
    n227 = Fract/Exp String To Number(string=w417) -> (number=w192:dbl)  [unwired: 3 in, 1 out]
    n228 = Fract/Exp String To Number(string=w378) -> (number=w191:dbl)  [unwired: 3 in, 1 out]
    n229 = Fract/Exp String To Number(string=w411) -> (number=w211:dbl)  [unwired: 3 in, 1 out]
    "TC 1" <- w211
    "TC1" <- w211
    n230 = Fract/Exp String To Number(string=w410) -> (number=w210:dbl)  [unwired: 3 in, 1 out]
    "TC 2" <- w210
    "TC2" <- w210
    n231 = Fract/Exp String To Number(string=w409) -> (number=w209:dbl)  [unwired: 3 in, 1 out]
    "TC 3" <- w209
    "TC3" <- w209
    n232 = Equal?(x=w321, y=w201) -> (x = y?=w323:bool)
    n233 = Equal?(x=w370, y="String 3") -> (x = y?=→"?":bool)
    n234 = Multiply(x=w197, y=w235) -> (x*y=w242:dbl)
    n235 = Multiply(x=w196, y=w233) -> (x*y=w241:dbl)
    n236 = Multiply(x=w195, y=w231) -> (x*y=w240:dbl)
    n237 = Multiply(x=w194, y=w229) -> (x*y=w239:dbl)
    n238 = Multiply(x=w193, y=w227) -> (x*y=w238:dbl)
    n239 = Multiply(x=w192, y=w224) -> (x*y=w237:dbl)
    n240 = Index Array(array=w271, index=w269) -> (element=w274:string)
    n241 = Fract/Exp String To Number(string=w401) -> (number=w184:dbl)  [unwired: 3 in, 1 out]
    n242 = Fract/Exp String To Number(string=w316) -> (number=w207:dbl)  [unwired: 3 in, 1 out]
    "Motor 1" <- w207
    n243 = Fract/Exp String To Number(string=w314) -> (number=w312:dbl)  [unwired: 3 in, 1 out]
    "Motor 3" <- w312
    n244 = Fract/Exp String To Number(string=w315) -> (number=w206:dbl)  [unwired: 3 in, 1 out]
    "Motor 2" <- w206
    n245 = Fract/Exp String To Number(string=w313) -> (number=w205:dbl)  [unwired: 3 in, 1 out]
    "Motor 4" <- w205
    n246 = Fract/Exp String To Number(string=w407) -> (number=w208:dbl)  [unwired: 3 in, 1 out]
    "TC 4" <- w208
    "TC4" <- w208
    n247 = Fract/Exp String To Number(string=w406) -> (number=w176:dbl)  [unwired: 3 in, 1 out]
    "TC 5" <- w176
    "TC5" <- w176
    n248 = Fract/Exp String To Number(string=w405) -> (number=w177:dbl)  [unwired: 3 in, 1 out]
    "TC 6" <- w177
    "TC6" <- w177
    n249 = Search/Split String(string=w201, search string/char (-)="r") -> (offset of match=w259:i32)  [unwired: 1 in, 2 out]
    n250 = Search/Split String(string=w201, search string/char (-)="z") -> (offset of match=w261:i32)  [unwired: 1 in, 2 out]
    n251 = Search/Split String(string=w201, search string/char (-)="s") -> (offset of match=w263:i32)  [unwired: 1 in, 2 out]
    n252 = Search/Split String(string=w201, search string/char (-)="a") -> (offset of match=w266:i32)  [unwired: 1 in, 2 out]
    n253 = Search/Split String(string=w201, search string/char (-)="t") -> (offset of match=w255:i32)  [unwired: 1 in, 2 out]
    n254 = Search/Split String(string=w201, search string/char (-)="e") -> (offset of match=w327:i32)  [unwired: 1 in, 2 out]
    n255 = local read "Manual Abort Tested"() -> (w256:bool)
    n256 = local read "Reset Triggered 2"() -> (w257:bool)
    n257 = local read "Multiplier 7"() -> (w222:dbl)
    n258 = case shown="False" w323 {
      tunnel: [w440 _] -> w322
      tunnel: w321 -> [w440 _]
      frame False {
      }
      frame True {
      }
    }
    n259 = Fract/Exp String To Number(string=w274) -> (number=→"ms":dbl)  [unwired: 3 in, 1 out]
    n260 = Greater Or Equal To 0?(x=w327) -> (x >= 0?=→"Craft Triggered Softkill Active":bool)
    n261 = Greater Or Equal To 0?(x=w266) -> (x >= 0?=w168:bool)
    "Hardkill Active" <- w168
    n262 = Greater Or Equal To 0?(x=w259) -> (x >= 0?=w185:bool)
    "Reset Triggered" <- w185
    n263 = Greater Or Equal To 0?(x=w261) -> (x >= 0?=w221:bool)
    "Flight Control On" <- w221
    n264 = Greater Or Equal To 0?(x=w255) -> (x >= 0?=w250:bool)
    "AV5-T Open" <- w250
    n265 = Greater Or Equal To 0?(x=w263) -> (x >= 0?=w251:bool)
    "Primary Safety Active" <- w251
    n266 = Equal?(x=w210, y=-2.0) -> (x = y?=→"gnd 2":bool)
    n267 = Equal?(x=w209, y=-2.0) -> (x = y?=→"gnd 3":bool)
    n268 = Equal?(x=w211, y=-1.0) -> (x = y?=→"TC1":bool)
    n269 = Equal?(x=w211, y=-2.0) -> (x = y?=→"gnd":bool)
    n270 = Equal?(x=w211, y=-3.0) -> (x = y?=→"vcc":bool)
    n271 = Equal?(x=w210, y=-1.0) -> (x = y?=→"TC2":bool)
    n272 = Equal?(x=w210, y=-3.0) -> (x = y?=→"vcc 2":bool)
    n273 = Equal?(x=w209, y=-1.0) -> (x = y?=→"TC3":bool)
    n274 = Equal?(x=w209, y=-3.0) -> (x = y?=→"vcc 3":bool)
    n275 = Multiply(x=w184, y=0.00488) -> (x*y=w182:dbl)
    n276 = Multiply(x=w191, y=w222) -> (x*y=w236:dbl)
    n277 = Or(x=w256, y=w168) -> (x .or. y?=w253:bool)
    "Manual Abort Tested" <- w253
    n278 = Or(x=w257, y=w185) -> (x .or. y?=w252:bool)
    "Reset Triggered 2" <- w252
    n279 = Bundle(w207, w206, w312, w205) -> (→"Motors":cluster{dbl, dbl, dbl, dbl})  [unwired: 1 in]
    n280 = Equal?(x=w208, y=-3.0) -> (x = y?=→"vcc 4":bool)
    n281 = Equal?(x=w176, y=-2.0) -> (x = y?=→"gnd 5":bool)
    n282 = Equal?(x=w208, y=-2.0) -> (x = y?=→"gnd 4":bool)
    n283 = Equal?(x=w208, y=-1.0) -> (x = y?=→"TC4":bool)
    n284 = Equal?(x=w176, y=-1.0) -> (x = y?=→"TC5":bool)
    n285 = Equal?(x=w176, y=-3.0) -> (x = y?=→"vcc 5":bool)
    n286 = Equal?(x=w177, y=-3.0) -> (x = y?=→"vcc 6":bool)
    n287 = Equal?(x=w177, y=-2.0) -> (x = y?=→"gnd 6":bool)
    n288 = Equal?(x=w177, y=-1.0) -> (x = y?=→"TC6":bool)
    n289 = Build Array(w253, w252, w221, w250, w251) -> (w249:bool[])
    n290 = Add(x=3.16, y=w182) -> (x+y=w180:dbl)
    n291 = local read "Offset 1"() -> (w234:dbl)
    n292 = local read "Offset 2"() -> (w232:dbl)
    n293 = local read "Offset 3"() -> (w230:dbl)
    n294 = local read "Offset 4"() -> (w228:dbl)
    n295 = local read "Offset 5"() -> (w226:dbl)
    n296 = local read "Offset 6"() -> (w225:dbl)
    n297 = local read "Offset 7"() -> (w223:dbl)
    n298 = And Array Elements(Boolean array=w249) -> (logical AND=w245:bool)
    "Ready to Test" <- w245
    n299 = Multiply(x=3.4776, y=w180) -> (x*y=w178:dbl)
    "Voltage Sensor" <- w178
    "?" <- w178
    n300 = case shown="True" "Send" {
      tunnel: w267 -> [_ w530]
      tunnel: w322 -> [_ w529]
      tunnel: w187 -> [_ w528]
      frame False {
      }
      frame True {
        n301 = case shown="No Error" w530 {
          selector: w530 -> [w533 w536]
          tunnel: [w535 _] -> _
          tunnel: [w534 w536] -> _
          tunnel: w529 -> [w532 _]
          tunnel: w528 -> [w531 _]
          frame No Error {
            n302 = VISA Write(VISA resource name=w531, write buffer=w532, error in (no error)=w533) -> (VISA resource name out=w535:refnum<visa-resource-name>, error out=w534:errorcluster)  [unwired: 1 out]
          }
          frame Error {
          }
        }
      }
    }
    n303 = And(x=w248, y=w245) -> (x .and. y?=w247:bool)
    n304 = Add(x=w234, y=w242) -> (x+y=w172:dbl)
    "PT 1" <- w172
    "PT4-M" <- w172
    n305 = Add(x=w232, y=w241) -> (x+y=w166:dbl)
    "PT 2" <- w166
    "PT1-M" <- w166
    n306 = Add(x=w230, y=w240) -> (x+y=w216:dbl)
    "PT 3" <- w216
    "PT3-M" <- w216
    n307 = Add(x=w228, y=w239) -> (x+y=w215:dbl)
    "PT 4" <- w215
    "PT1-U" <- w215
    n308 = Add(x=w226, y=w238) -> (x+y=w214:dbl)
    "PT 5" <- w214
    "PT2-U" <- w214
    n309 = Add(x=w225, y=w237) -> (x+y=w213:dbl)
    "PT 6" <- w213
    "PT2-M" <- w213
    n310 = Add(x=w223, y=w236) -> (x+y=w212:dbl)
    "PT5-M" <- w212
    "PT 7" <- w212
    n311 = Or(x=w248, y=w247) -> (x .or. y?=w246:bool)
    n312 = Exclusive Or(1:w246, 2:"Begin Checklist") -> (0:w264:bool)
    n313 = Build Array(w197, w196, w195, w194, w193, w192, w191, w172, w166, w216, w215, w214, w213, w212, w211, w210, w209, w208, w176, w177, w178, w207, w206, w206, w205) -> (w204:dbl[])
    n314 = Bundle(w178, w211, w210, w209, w208, w176, w177, w172, w166, w216, w215, w214, w213, w212) -> (w188:T1)  [unwired: 1 out]
    "?" <- w188
    n315 = case shown="True" w264 {
      frame False {
      }
      frame True {
        w439 = FALSE
        n316 = local write "Reset Triggered 2"(w439) -> ()
        n317 = local write "Manual Abort Tested"(w439) -> ()
      }
    }
    n318 = Array To Spreadsheet String(delimiter (Tab)="\t", array=w204, 3:"%d" ("format string")) -> (spreadsheet string=w175:string)
    n319 = Max & Min(x=w189, y=w188) -> (max(x,y)=w190:T1)  [unwired: 1 out]
    "Max Values" <- w190
    n320 = Search/Split String(string=w175, search string/char (-)="\r\n") -> (substring before match=w173:string)  [unwired: 1 in, 2 out]
    n321 = Concatenate Strings(w173, "\t" ("string"), w201, "\n" ("string")) -> (w199:string)
    n322 = Write to Text File(file (use dialog)=w220, text=w199) -> (refnum out=w217:refnum<file>)  [unwired: 2 in, 2 out]
    "FO-U" <- "FOU"
    "AV5-T" <- "tank iso"
    "FC-U" <- "FC-U Toggle"
    "Numeric" <- w159
  }
  n323 = VISA Close(VISA resource name=w1, error in (no error)=w56) -> ()  [unwired: 1 out]
  n324 = Close File(refnum=w52) -> ()  [unwired: 1 in, 2 out]
